vi "CreateDirs.vi"(8 "error in (no error)":errorcluster, 11 "Shell Arguments":T2) -> (0 "error out":errorcluster, 3 "Output Folders":T1)   [LabVIEW 2020, in "VIDiffUtilities.lvlib"]
uses:
  VIDiffUtilities.lvlib
  Arguments.ctl
  Output Folders.ctl
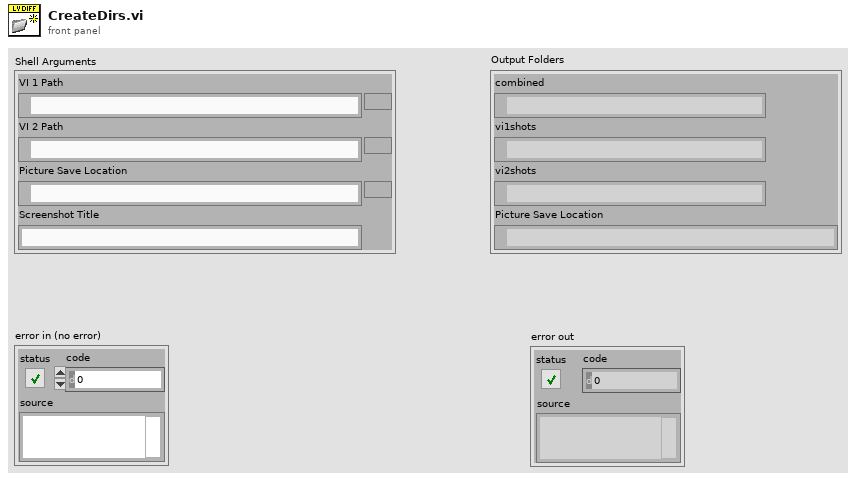
[diagram p1: front panel]
types:
  T1 = typedef "VIDiffUtilities.lvlib/Output Folders.ctl" = cluster{"combined":path, "vi1shots":path, "vi2shots":path, "Picture Save Location":path}
  T2 = typedef "VIDiffUtilities.lvlib/Arguments.ctl" = cluster{"VI 1 Path":path, "VI 2 Path":path, "Picture Save Location":path, "Screenshot Title":string}
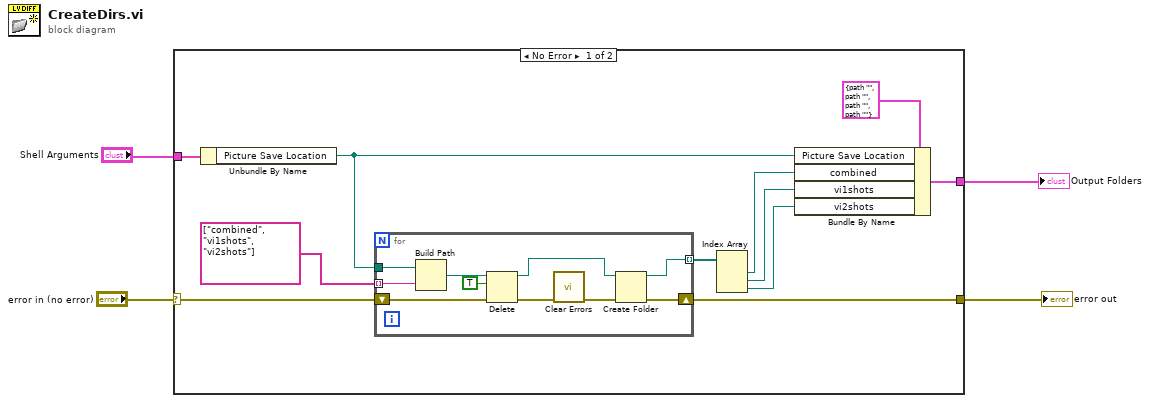
[diagram p0: block diagram]
diagram:
  n1 = case shown="No Error" "error in (no error)" {
    selector: "error in (no error)" -> [w13 w26]
    tunnel: [w12 w26] -> w3
    tunnel: "Shell Arguments" -> [w15 _]
    tunnel: [w6 _] -> w1
    frame No Error {
      n2 = Unbundle By Name(w15) -> ("Picture Save Location"=w5:path)
      n3 = for {
        tunnel: w5 -> [w20]
        tunnel: string[] ["combined", "vi1shots", "vi2shots"] -> [w19] mode=indexing
        shift-right: [w18] -> w12
        shift-left: w13 -> [w17]
        tunnel: [w16] -> w11 mode=indexing
        n4 = Build Path(base path=w20, name or relative path=w19) -> (appended path=w25:path)
        n5 = Delete(path (use dialog)=w25, entire hierarchy (F)=TRUE, error in=w17) -> (deleted path=w24:path, error out=w23:errorcluster)  [unwired: 2 in, 1 out]
        n6 = call <vilib>:"Clear Errors.vi"("error in (no error)"=w23) -> ("error out"=w22:errorcluster)  [unwired: 5 in, 1 out]
        n7 = Create Folder(path (use dialog)=w24, error in=w22) -> (created path=w16:path, error out=w18:errorcluster)  [unwired: 1 in, 1 out]
      }
      n8 = Index Array(array=w11) -> (element #1=w9:path, element #2=w8:path, element #3=w7:path)  [unwired: 3 in]
      n9 = Bundle By Name(cluster=T1 {"combined"=path "", "vi1shots"=path "", "vi2shots"=path "", "Picture Save Location"=path ""} ("Output Folders"), "Picture Save Location"=w5, "combined"=w9, "vi1shots"=w8, "vi2shots"=w7) -> (w6:T1)
    }
    frame Error {
    }
  }
  "error out" <- w3
  "Output Folders" <- w1
